vi "בדיקת זמן ניתוק הממסר 7.vi"(7 "resultUserPrompt":bool, 8 "error":errorcluster, 11 "Path for Log":path) -> (0 "error out":errorcluster, 1 "בטוח כן/לא":bool, 2 "בדיקת זמן ניתוק הממסר":dbl)   [LabVIEW 2015]
uses:
  <instrlib>/niDMM/nidmm.llb/niDMM Function.ctl
  <instrlib>/niDMM/nidmm.llb/niDMM Resolution in Digits.ctl
  <vilib>/DAQmx/write.llb/DAQmx Write (Digital Bool 1Line 1Point).vi
  <vilib>/DAQmx/create/channels.llb/DAQmx Create Channel (DO-Digital Output).vi
  <vilib>/DAQmx/miscellaneous.llb/DAQmx Fill In Error Info.vi
  <instrlib>/niDMM/nidmm.llb/niDMM Configure Measurement Digits.vi
panel:
  # "Right-Click to\nexplain error"
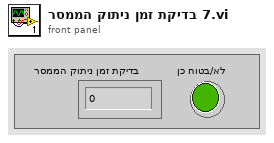
[diagram p1: front panel]
types:
  T1 = enum32{"Invalid", "Standard", "Closed", "Hidden", "Minimized", "Maximized"}
  T2 = typedef "niDMM Function.ctl" = enum16{"DC Volts", "AC Volts", "DC Current", "AC Current", "2-wire Resistance", "4-wire Resistance", "Diode", "Frequency", "Period", "AC Volts DC Coupled", "Capacitance", "Inductance", "Temperature"}
  T3 = typedef "niDMM Resolution in Digits.ctl" = dbl
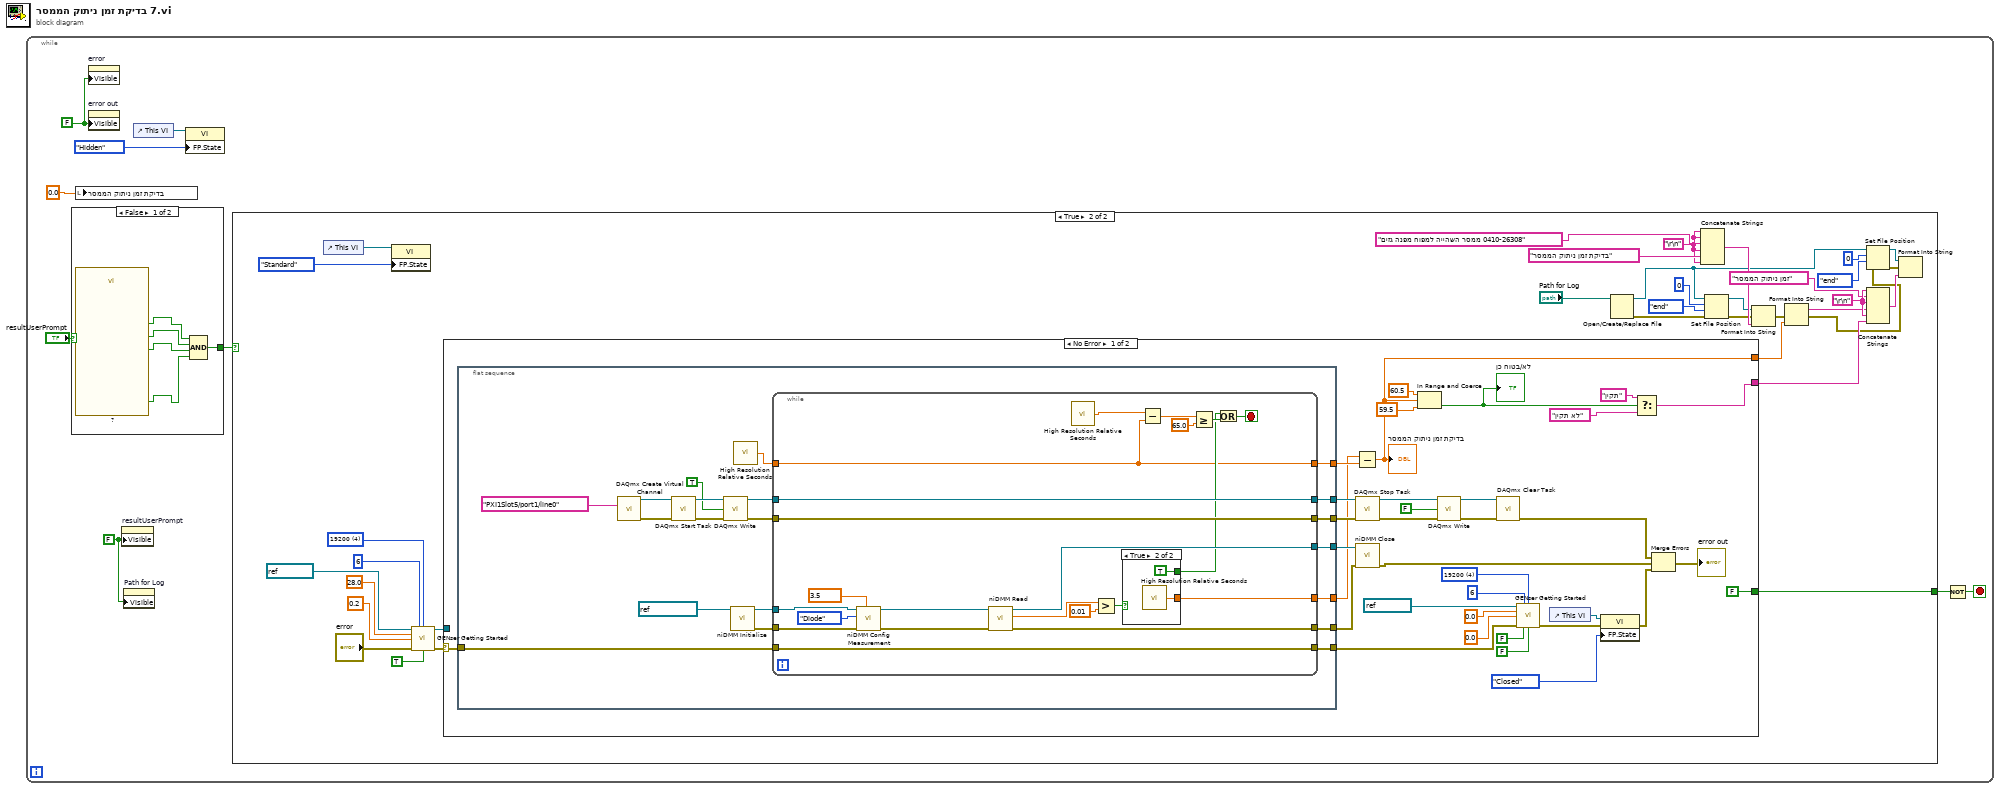
[diagram p0: block diagram]
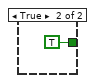
[diagram p2: hidden frame]
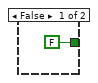
[diagram p3: hidden frame]
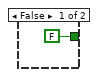
[diagram p4: hidden frame]
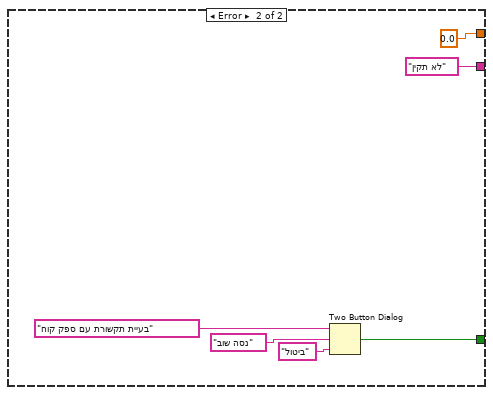
[diagram p5: hidden frame]
diagram:
  n1 = while {
    stop <- w8 stop-if-true
    w1 = FALSE ("Visible")
    w6 = FALSE ("Visible")
    n2 = case shown="False" "resultUserPrompt" {
      tunnel: [w14 TRUE] -> w9
      frame False {
        n3 = call "?"() -> ("הדקי הרב מודד"=w10:bool, "(מגע שלילי (מעטפת"=w11:bool, "C מגע חיובי"=w12:bool, "OK"=w13:bool)  [unwired: 15 in, 1 out]
        n4 = Compound Arithmetic op=AND(w13, w12, w11, w10) -> (w14:bool)
      }
      frame True {
      }
    }
    n5 = local write "בדיקת זמן ניתוק הממסר"(0.0 ("זמן ניתוק הממסר")) -> ()
    n6 = property on="error" class="Clust (strict)"("Visible"=w6) -> ()  [unwired: 2 in, 2 out]
    n7 = property on="error out" class="Clust (strict)"("Visible"=w6) -> ()  [unwired: 2 in, 2 out]
    n8 = property on="resultUserPrompt" class="Bool (strict)"("Visible"=w1) -> ()  [unwired: 2 in, 2 out]
    n9 = property on="Path for Log" class="Path"("Visible"=w1) -> ()  [unwired: 2 in, 2 out]
    n10 = control-ref of="This VI"() -> (w5:refnum<vi>)
    n11 = property class="VI"(reference=w5, "FP.State"=T1."Hidden" ("Front Panel Window:State")) -> ()  [unwired: 1 in, 2 out]
    n12 = case shown="True" w9 {
      tunnel: [FALSE ("T button?") w44] -> w7
      frame False {
      }
      frame True {
        w26 = "\r\n"
        w34 = "\r\n"
        w48 = u16 4 items=["1200", "2400", "4800", "9600", "19200"] ("BAUD")
        n13 = control-ref of="This VI"() -> (w43:refnum<vi>)
        n14 = property class="VI"(reference=w43, "FP.State"=T1."Standard" ("Front Panel Window:State")) -> ()  [unwired: 1 in, 2 out]
        n15 = call "GENser Getting Started.vi"("VISA"=refnum<visa-resource-name> "COM6", "GEN Addr"=i16 6, "BAUD"=w48, "Voltage Limit"=28.0, "Current Limit"=0.2, "error"="error", "Output On (T)"=TRUE) -> ("VISA out"=w49:refnum<visa-resource-name>, "error out"=w40:errorcluster)  [unwired: 5 in, 2 out]
        n16 = case shown="No Error" w40 {
          selector: w40 -> [w78 _]
          tunnel: w49 -> [_ _]
          tunnel: [FALSE ("T button?") w134] -> w44
          tunnel: [w56 0.0] -> w20
          tunnel: [w52 "לא תקין"] -> w19
          frame No Error {
            w73 = u16 4 items=["1200", "2400", "4800", "9600", "19200"] ("BAUD")
            n17 = flat-sequence {
              tunnel: [w100] -> w57
              tunnel: [w99] -> w58
              tunnel: [w98] -> w65
              tunnel: [w97] -> w66
              tunnel: [w96] -> w62
              tunnel: w78 -> [w95]
              tunnel: [w94] -> w77
              tunnel: [w93] -> w63
              frame #0 {
                n18 = call-poly <vilib>:"DAQmx Create Virtual Channel.vi"("lines"=tag "PXI1Slot5/port1/line0") -> ("task out"=w102:refnum<k21>, "error out"=w103:errorcluster)  [unwired: 13 in]
                n19 = call <vilib>:"DAQmx Start Task.vi"("task/channels in"=w102, "error in"=w103) -> ("task out"=w92:refnum<k21>, "error out"=w91:errorcluster)  [unwired: 12 in]
                n20 = call-poly <vilib>:"DAQmx Write.vi"("task/channels in"=w92, "data"=TRUE, "error in"=w91) -> ("task out"=w89:refnum<k21>, "error out"=w90:errorcluster)  [unwired: 10 in, 1 out]
                n21 = call <instrlib>:"niDMM Initialize.vi"("Instrument Descriptor"=refnum<k15> "PXI1Slot9") -> ("error out"=w104:errorcluster, "instrument handle out"=w105:refnum<k15>)  [unwired: 9 in]
                n22 = call <vilib>:"High Resolution Relative Seconds.vi"() -> ("relative seconds"=w87:dbl)
                n23 = while {
                  tunnel: [w108] -> w99
                  tunnel: [w126] -> w100
                  tunnel: [w119] -> w96
                  tunnel: [w111] -> w97
                  tunnel: [w110] -> w98
                  tunnel: [w118] -> w93
                  tunnel: w105 -> [w123]
                  tunnel: w104 -> [w122]
                  tunnel: w89 -> [w111]
                  tunnel: w90 -> [w110]
                  tunnel: [w112] -> w94
                  tunnel: w95 -> [w112]
                  tunnel: w87 -> [w108]
                  stop <- w115 stop-if-true
                  w128 = T3 3.5 items=["3 1/2"=3.5, "4 1/2"=4.5, "5 1/2"=5.5, "6 1/2"=6.5, "7 1/2"=7.5] ("Resolution in Digits")
                  n24 = call-poly <instrlib>:"niDMM Config Measurement.vi"("Resolution in Digits"=w128, "error in (no error)"=w122, "Function"=niDMM_Function."Diode", "instrument handle"=w123) -> ("error out"=w120:errorcluster, "instrument handle out"=w121:refnum<k15>)  [unwired: 6 in]
                  n25 = call <instrlib>:"niDMM Read.vi"("error in (no error)"=w120, "instrument handle"=w121) -> ("error out"=w118:errorcluster, "Measurement"=w125:dbl, "instrument handle out"=w119:refnum<k15>)  [unwired: 7 in]
                  n26 = call <vilib>:"High Resolution Relative Seconds.vi"() -> ("relative seconds"=w107:dbl)
                  n27 = Greater?(x=w125, y=0.01) -> (0:w113:bool)
                  n28 = case shown="True" w113 {
                    tunnel: [_ w131] -> w126
                    tunnel: [FALSE TRUE] -> w109
                    frame False {
                    }
                    frame True {
                      n29 = call <vilib>:"High Resolution Relative Seconds.vi"() -> ("relative seconds"=w131:dbl)
                    }
                  }
                  n30 = Subtract(x=w107, y=w108) -> (x-y=w117:dbl)
                  n31 = Greater Or Equal?(x=w117, y=65.0) -> (x >= y?=w114:bool)
                  n32 = Or(x=w109, y=w114) -> (x .or. y?=w115:bool)
                }
              }
            }
            n33 = Subtract(x=w57, y=w58) -> (x-y=w56:dbl)
            "בדיקת זמן ניתוק הממסר" <- w56
            n34 = call <vilib>:"DAQmx Stop Task.vi"("task/channels in"=w66, "error in"=w65) -> ("task out"=w71:refnum<k21>, "error out"=w70:errorcluster)  [unwired: 12 in]
            n35 = call <instrlib>:"niDMM Close.vi"("error in (no error)"=w63, "instrument handle"=w62) -> ("error out"=w61:errorcluster)  [unwired: 9 in]
            n36 = In Range and Coerce(upper limit=60.5, x=w56, lower limit=59.5) -> (In Range?=w53:bool)  [unwired: 1 out]
            "בטוח כן/לא" <- w53
            n37 = call-poly <vilib>:"DAQmx Write.vi"("task/channels in"=w71, "data"=FALSE, "error in"=w70) -> ("task out"=w68:refnum<k21>, "error out"=w69:errorcluster)  [unwired: 10 in, 1 out]
            n38 = call <vilib>:"DAQmx Clear Task.vi"("task in"=w68, "error in"=w69) -> ("error out"=w64:errorcluster)  [unwired: 13 in]
            n39 = call "GENser Getting Started.vi"("VISA"=refnum<visa-resource-name> "COM6", "GEN Addr"=i16 6, "BAUD"=w73, "Voltage Limit"=0.0, "Current Limit"=0.0, "error"=w77, "Reset (T)"=FALSE ("Output On (T)"), "Output On (T)"=FALSE) -> ("error out"=w79:errorcluster)  [unwired: 4 in, 3 out]
            n40 = control-ref of="This VI"() -> (w81:refnum<vi>)
            n41 = property class="VI"(reference=w81, error in=w79, "FP.State"=T1."Closed" ("Front Panel Window:State")) -> (error out=w75:errorcluster)  [unwired: 1 out]
            n42 = Select(t="תקין", s=w53, f="לא תקין") -> (s? t:f=w52:string)
            n43 = Merge Errors(w64, w61, w75) -> (→"error out":errorcluster)
          }
          frame Error {
            n44 = Two Button Dialog(message="בעיית תקשורת עם ספק קוח", 1:"ביטול" ("F button name (\"Cancel\")"), 2:"נסה שוב" ("T button name (\"OK\")")) -> (T button?=w134:bool)
          }
        }
        n45 = Open/Create/Replace File(file path (use dialog)="Path for Log") -> (refnum out=w21:refnum<file>, error out=w22:errorcluster)  [unwired: 5 in, 1 out]
        n46 = Concatenate Strings(w34, w34, "ממסר השהייה למפוח מפנה גזים 0410-26308", w34, "בדיקת זמן ניתוק הממסר", w34) -> (w37:string)
        n47 = Set File Position(offset (in bytes) (0)=i64 0, refnum=w21, from (0:start)=enum16{"start", "end", "current"}."end", error in=w22) -> (refnum out=w35:refnum<file>, error out=w33:errorcluster)
        n48 = Format Into String(initial string=w35, error in=w33, w37) -> (error out=w32:errorcluster)  [unwired: 1 in, 1 out]
        n49 = Format Into String(error in=w32, w20) -> (resulting string=w24:string, error out=w18:errorcluster)  [unwired: 2 in]
        n50 = Set File Position(offset (in bytes) (0)=i64 0, refnum=w21, from (0:start)=enum16{"start", "end", "current"}."end", error in=w18) -> (refnum out=w29:refnum<file>, error out=w30:errorcluster)
        n51 = Concatenate Strings(w26, "זמן ניתוק הממסר", w26, w24, w26, w19) -> (w31:string)
        n52 = Format Into String(initial string=w29, error in=w30, w31) -> ()  [unwired: 1 in, 2 out]
      }
    }
    n53 = Not(x=w7) -> (.not. x?=w8:bool)
  }
